vi "P2_2_Temperaturas.vi"() -> ()   [LabVIEW 2020]
panel:
  out "Arreglo Unido de Temperaturas":dbl[][](array[numeric])
  out "min value":dbl
  out "max value":dbl
  out "Waveform Graph 2":dbl[](graph)
  out "Waveform Graph":dbl[](graph)
  out "Array 3":dbl[](array[numeric])
  out "Array 2":dbl[](array[numeric])
  out "Array":dbl[](array[numeric])
  # "C°"
  # "F°"
  # "EMA"
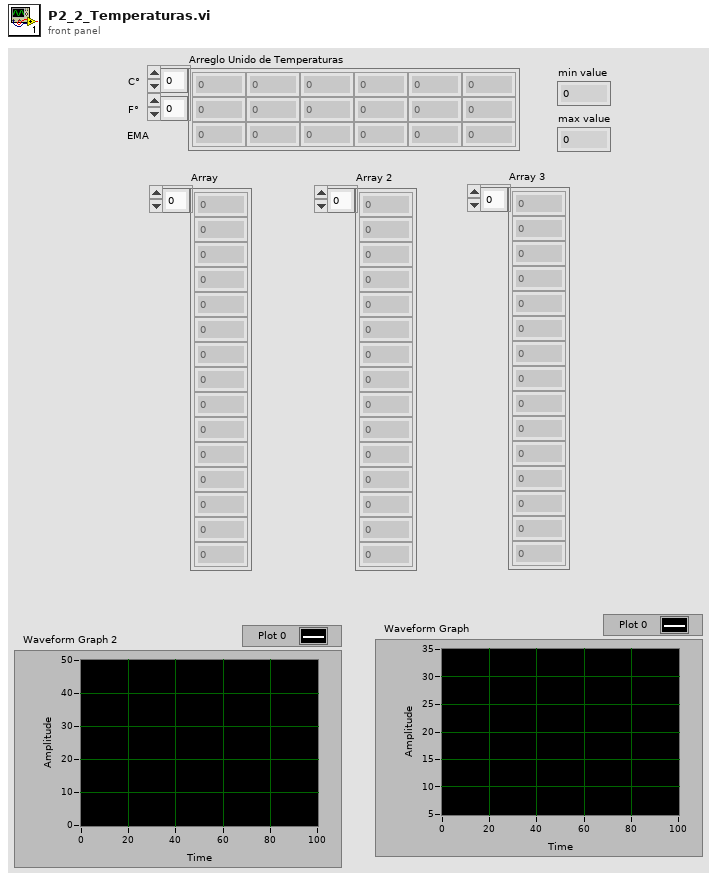
[diagram p1: front panel]
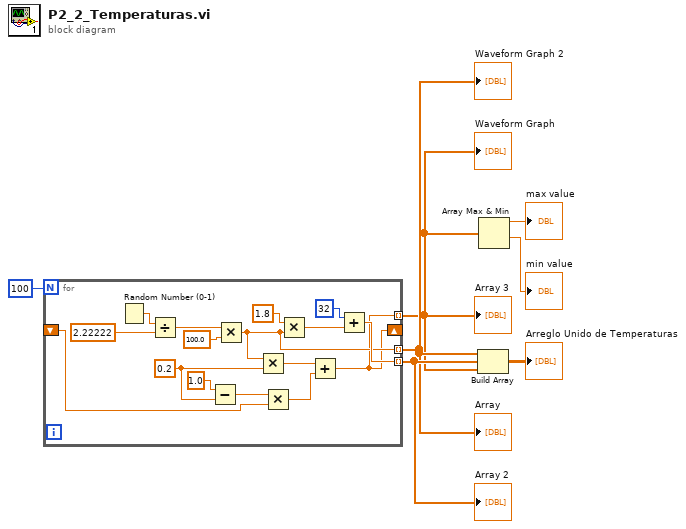
[diagram p0: block diagram]
diagram:
  n1 = for {
    N: 100 -> [_]
    tunnel: [w15] -> w5 mode=indexing
    tunnel: [w16] -> w6 mode=indexing
    shift-right: [w9] -> _
    shift-left: _ -> [w8]
    tunnel: [w9] -> w2 mode=indexing
    w13 = 0.2
    n2 = Random Number (0-1)() -> (number: 0 to 1=w23:dbl)
    n3 = Divide(x=w23, y=2.22222) -> (x/y=w20:dbl)
    n4 = Subtract(x=1.0, y=w13) -> (x-y=w11:dbl)
    n5 = Multiply(x=w20, y=100.0 ("x*y")) -> (x*y=w15:dbl)
    n6 = Multiply(x=w15, y=w13) -> (x*y=w10:dbl)
    n7 = Multiply(x=w11, y=w8) -> (x*y=w12:dbl)
    n8 = Multiply(x=1.8, y=w15) -> (x*y=w18:dbl)
    n9 = Add(x=w10, y=w12) -> (x+y=w9:dbl)
    n10 = Add(x=32, y=w18) -> (x+y=w16:dbl)
  }
  "Array" <- w5
  "Array 2" <- w6
  "Array 3" <- w2
  "Waveform Graph" <- w2
  "Waveform Graph 2" <- w5
  n11 = Build Array(w5, w6, w2) -> (→"Arreglo Unido de Temperaturas":dbl[][])
  n12 = Array Max & Min(array=w2) -> (max value=→"max value":dbl, min value=→"min value":dbl)  [unwired: 2 out]
